vi "Layout - Insert Layout-VI into SP_Main.vi"(7 "SubPanel in":refnum<vi>, 8 "error in (no error)":errorcluster, 11 "Layout-VI Ref":refnum<vi>) -> (0 "error out":errorcluster)   [LabVIEW 2022 SP3, in "UI Manager.lvlib"]
doc: "Inserts the Layout-VI via its reference into the SP_Main subpanel on the UI Manager frontpanel.\n\n____\nHAMPEL SOFTWARE ENGINEERING v2.6.0 (2023-12-19 10:54)"
uses:
  UI Manager.lvlib
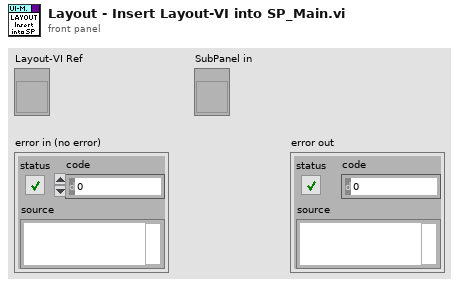
[diagram p1: front panel]
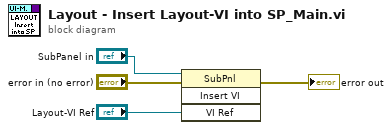
[diagram p0: block diagram]
diagram:
  n1 = invoke class="SubPnl" method="Insert VI"(reference="SubPanel in", error in="error in (no error)", "VI Ref"="Layout-VI Ref") -> (error out=→"error out":errorcluster)  [unwired: 1 in, 3 out]
